vi "startUp.vi"(8 "error in (no error)":errorcluster, 11 "CameraControlViewer in":refnum<class "CameraControlViewer.lvclass">) -> (0 "error out":errorcluster, 3 "CameraControlViewer out":refnum<class "CameraControlViewer.lvclass">)   [LabVIEW 2011, in "Views.lvlib" / "Camera.lvlib" / "CameraControlViewer.lvclass"]
uses:
  CameraControlViewer.lvclass
  CameraControlViewer.lvclass/CameraControlViewer.ctl
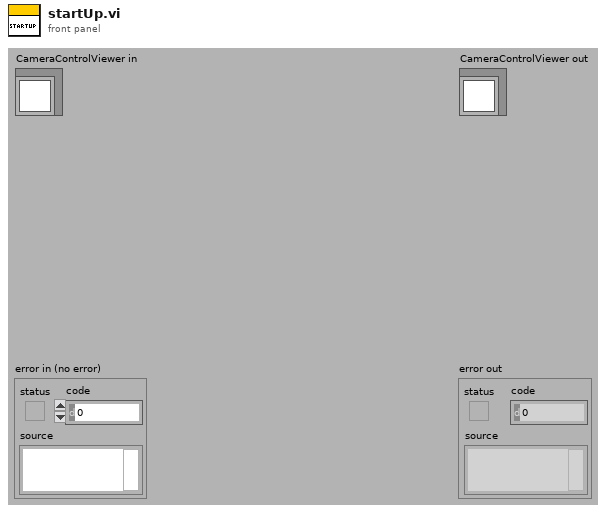
[diagram p1: front panel]
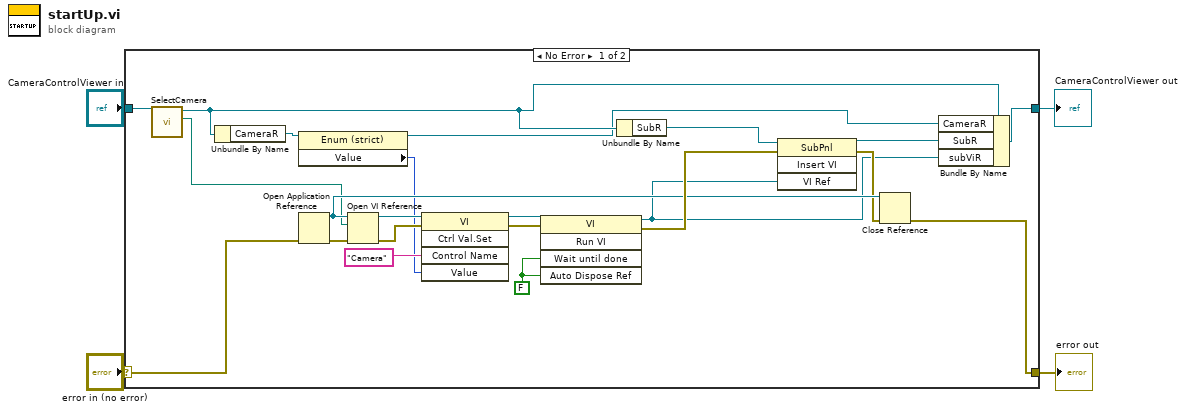
[diagram p0: block diagram]
diagram:
  n1 = case shown="No Error" "error in (no error)" {
    selector: "error in (no error)" -> [w24 w28]
    tunnel: [w17 w28] -> w3
    tunnel: [w19 w27] -> w1
    tunnel: "CameraControlViewer in" -> [w14 w27]
    frame No Error {
      w26 = FALSE
      n2 = call "SelectCamera.vi"("CameraControlViewer in"=w14) -> ("CameraSettingsPath"=w13:path, "CameraControlViewer out"=w8:refnum<class "CameraControlViewer.lvclass">)  [unwired: 8 in, 1 out]
      n3 = Unbundle By Name(w8) -> ("CameraR"=w7:refnum<vi>)
      n4 = property class="Enum (strict)"(reference=w7) -> (reference out=w5:refnum<vi>, "Value"=w6:enum16{"Pixis", "ProEM", "PixelFly"})  [unwired: 1 in, 1 out]
      n5 = Open Application Reference(8:w24) -> (0:w25:errorcluster, 3:w21:refnum<vi>)  [unwired: 3 in]
      n6 = Open VI Reference(application reference (local)=w21, vi path=w13, error in (no error)=w25) -> (vi reference=w16:refnum<vi>, error out=w11:errorcluster)  [unwired: 3 in]
      n7 = invoke class="VI" method="Ctrl Val.Set"(reference=w16, error in=w11, "Control Name"="Camera", "Value"=w6) -> (reference out=w12:refnum<vi>, error out=w10:errorcluster)  [unwired: 1 in, 3 out]
      n8 = invoke class="VI" method="Run VI"(reference=w12, error in=w10, "Wait until done"=w26, "Auto Dispose Ref"=w26) -> (reference out=w15:refnum<vi>, error out=w22:errorcluster)  [unwired: 1 in, 3 out]
      n9 = Unbundle By Name(w8) -> ("SubR"=w23:refnum<vi>)
      n10 = invoke class="SubPnl" method="Insert VI"(reference=w23, error in=w22, "VI Ref"=w15) -> (reference out=w18:refnum<vi>, error out=w20:errorcluster)  [unwired: 1 in, 2 out]
      n11 = Close Reference(reference=w21, error in (no error)=w20) -> (error out=w17:errorcluster)
      n12 = Bundle By Name(cluster=w8, "CameraR"=w5, "SubR"=w18, "subViR"=w15) -> (w19:refnum<class "CameraControlViewer.lvclass">)
    }
    frame Error {
    }
  }
  "error out" <- w3
  "CameraControlViewer out" <- w1
